vi "USRP Start Trigger.vi"(0 "stream enable":bool, 1 "trigger select":T1=enum."Immediate", 5 "trigger enable":bool, 7 "software trigger":bool, 9 "other start trigger":bool, 11 "event occurred":bool) -> (4 "start trigger":bool)   [LabVIEW 2016]
doc: "Generates start triggers for Rx and Tx. Start triggers are generated based on which trigger type is selected, whether the stream is enabled, whether triggers are enabled, and whether the triggers are to be synchronized across multiple devices.\n\n<B>Input Parameters</B>\n\n<B>enable stream</B> controls the output of a 'start trigger'.\n\n<B>software trigger</B> is a start trigger asserted by software.\n\n<B>enable trigger</B> controls the output of a 'start trigger'.\n\n<B>enable trigger sync</B> to synchronize a 'start trigger' between multiple devices. The master device sends the 'start trigger' to all the slave devices. If enabled, the slave devices ignore the 'trigger select' because the 'start trigger' from the master device is used instead.\n\n<B>trigger select</B> picks which source to use as the 'start trigger'.\n\n<B>Output Parameters</B>\n\n<B>rx.start trigger</B> is the signal to use at the 'start trigger' for the Rx data path.\n\n<B>tx.start trigger</B> is the signal to use at the 'start trigger' for the Tx data path."
uses:
  Host/SubVIs/USRP Start Trigger.ctl
  <vilib>/rvi/eio/common/nirviEmuTemplateMethod_errors.vi
  <vilib>/eio/EIONode/EIONode.xnode
  <instrlib>/_niInstr/Basic Elements/v1/FPGA/niInstr Basic Elements v1 FPGA.lvlib
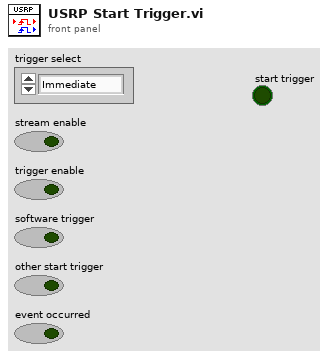
[diagram p1: front panel]
types:
  T1 = typedef "USRP Start Trigger.ctl" = enum8{"Software", "Digital Edge", "Rx Start Trigger", "Tx Start Trigger", "Immediate", "Future Time Event"}
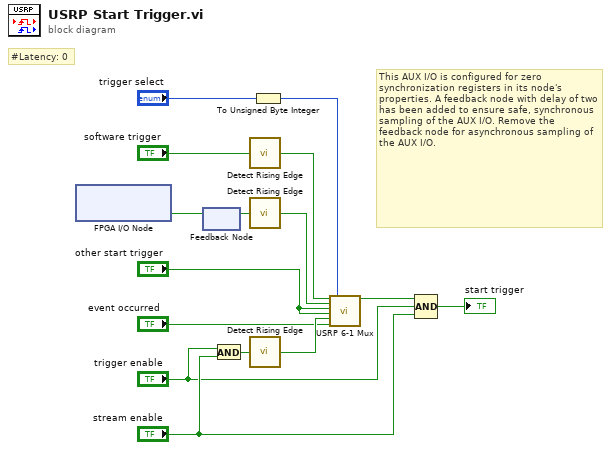
[diagram p0: block diagram]
diagram:
  # "#Latency: 0"
  # "This AUX I/O is configured for zero synchronization registers in its node's properties. A feedback node with delay of two has been added to ensure safe, synchronous sampling of the AUX I/O. Remove the feedback node for asynchronous sampling of the AUX I/O."
  n1 = xnode "FPGA I/O Node"() -> ("AUX I/O 0"=w11:bool)  [unwired: 1 in, 1 out]
  n2 = feedback-in #1(w11) -> ()
  n3 = feedback #1() -> (w6:bool)  [unwired: 1 in]
  n4 = And(x="trigger enable", y="stream enable") -> (x .and. y?=w10:bool)
  n5 = call <instrlib>:"Detect Rising Edge.vi"("signal"="software trigger") -> ("edge detected"=w15:bool)  [unwired: 14 in]
  n6 = call <instrlib>:"Detect Rising Edge.vi"("signal"=w6) -> ("edge detected"=w3:bool)  [unwired: 14 in]
  n7 = call <instrlib>:"Detect Rising Edge.vi"("signal"=w10) -> ("edge detected"=w14:bool)  [unwired: 14 in]
  n8 = To Unsigned Byte Integer(number="trigger select") -> (unsigned 8bit integer=w9:u8)
  n9 = call "USRP 6-1 Mux.vi"("input 0"=w15, "input 1"=w3, "input 2"="other start trigger", "input 3"="other start trigger", "input 4"=w14, "input 5"="event occurred", "select"=w9) -> ("output"=w1:bool)  [unwired: 12 in]
  n10 = Compound Arithmetic op=AND(w1, "trigger enable", "stream enable") -> (→"start trigger":bool)
